vi "List Available Templates.vi"(8 "error in (no error)":errorcluster, 11 "ctl in":refnum<class "ctl.lvclass">) -> (0 "error out":errorcluster, 1 "Templates Paths":path[](array[path]), 2 "Templates Available":string[](array[string]), 3 "ctl out":refnum<class "ctl.lvclass">)   [LabVIEW 2012, in "ctl.lvclass"]
uses:
  ctl.lvclass
  ctl.lvclass/ctl.ctl
  <userlib>/_OpenG.lib/file/file.llb/Build Path - File Names Array__ogtk.vi
  <userlib>/_OpenG.lib/file/file.llb/Strip Path Extension - 1D Array of Strings__ogtk.vi
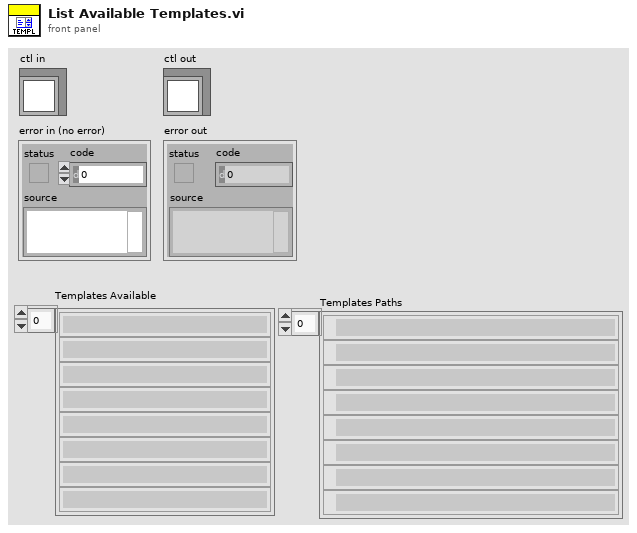
[diagram p1: front panel]
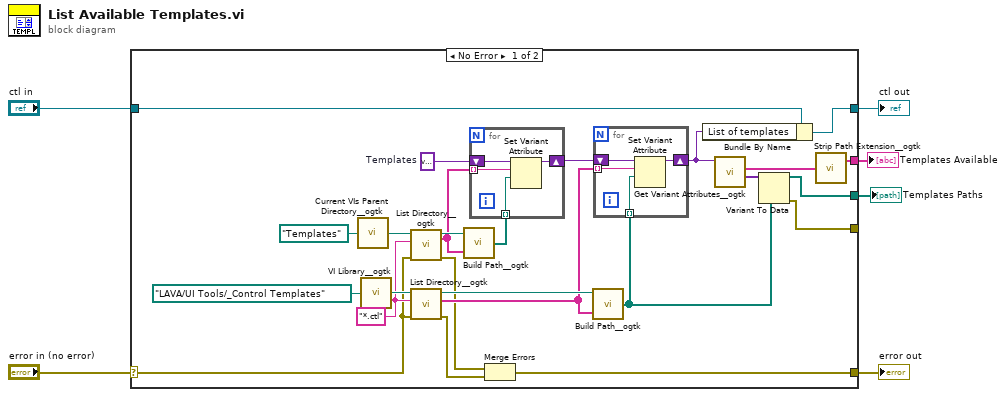
[diagram p0: block diagram]
diagram:
  n1 = case shown="No Error" "error in (no error)" {
    selector: "error in (no error)" -> [w27 w41]
    tunnel: [w8 w41] -> w5
    tunnel: [w11 w40] -> w3
    tunnel: "ctl in" -> [w12 w40]
    tunnel: [w16 _] -> w2
    tunnel: [w15 _] -> w1
    tunnel: [w7 _] -> _
    frame No Error {
      w26 = variant  # Templates
      w28 = "*.ctl" ("pattern")
      n2 = call <userlib>:"Current VIs Parent Directory__ogtk.vi"("Relative path (.)"=path "Templates") -> ("Parent Directory (+ Relative)"=w29:path)  [unwired: 4 in]
      n3 = call <userlib>:"VI Library__ogtk.vi"("Relative path (.)"=path "LAVA/UI Tools/_Control Templates") -> ("VI Library (+ Relative)"=w30:path)
      n4 = call <userlib>:"List Directory__ogtk.vi"("error in (no error)"=w27, "pattern"=w28, "directory path"=w29) -> ("error out"=w10:errorcluster, "file names"=w24:string[], "dup directory path"=w25:path)  [unwired: 1 in, 1 out]
      n5 = call <userlib>:"List Directory__ogtk.vi"("error in (no error)"=w27, "pattern"=w28, "directory path"=w30) -> ("error out"=w9:errorcluster, "file names"=w20:string[], "dup directory path"=w21:path)  [unwired: 1 in, 1 out]
      n6 = call-poly <userlib>:"Build Path__ogtk.vi"("name or relative path"=w24, "base path"=w25) -> ("appended path"=w23:path[])
      n7 = for {
        tunnel: w24 -> [w38] mode=indexing
        tunnel: w23 -> [w37] mode=indexing
        shift-right: [w36] -> w22
        shift-left: w26 -> [w39]
        n8 = Set Variant Attribute(Variant=w39, name=w38, value=w37) -> (Variant out=w36:variant)  [unwired: 1 in, 2 out]
      }
      n9 = Merge Errors(w10, w9) -> (w8:errorcluster)
      n10 = call-poly <userlib>:"Build Path__ogtk.vi"("name or relative path"=w20, "base path"=w21) -> ("appended path"=w18:path[])
      n11 = for {
        tunnel: w20 -> [w34] mode=indexing
        tunnel: w18 -> [w33] mode=indexing
        shift-right: [w32] -> w13
        shift-left: w22 -> [w35]
        n12 = Set Variant Attribute(Variant=w35, name=w34, value=w33) -> (Variant out=w32:variant)  [unwired: 1 in, 2 out]
      }
      n13 = Bundle By Name(cluster=w12, "List of templates"=w13) -> (w11:refnum<class "ctl.lvclass">)
      n14 = call <userlib>:"Get Variant Attributes__ogtk.vi"("Variant"=w13) -> ("value(s)"=w19:variant[], "names"=w17:string[])  [unwired: 3 in, 2 out]
      n15 = Variant To Data(type=w18, Variant=w19) -> (data=w15:path[], error out=w7:errorcluster)  [unwired: 1 in]
      n16 = call-poly <userlib>:"Strip Path Extension__ogtk.vi"("paths"=w17) -> ("roots"=w16:string[])  [unwired: 1 out]
    }
    frame Error {
    }
  }
  "error out" <- w5
  "ctl out" <- w3
  "Templates Available" <- w2
  "Templates Paths" <- w1
